vi "LvMPDC_CMD_Playlist_delete.vi"(6 "timeout_ms":i32=3000, 8 "error in (no error)":errorcluster, 9 "ReadBytes":i32=1024, 10 "pos":i32=-1, 11 "Connect ID":refnum<k5>) -> (0 "error out":errorcluster, 3 "Connect ID out":refnum<k5>)   [LabVIEW 2012]
panel:
  # "LvMPDC:: CMD delete (delete from Playlist)"
  # "-1 は番号指定無し"
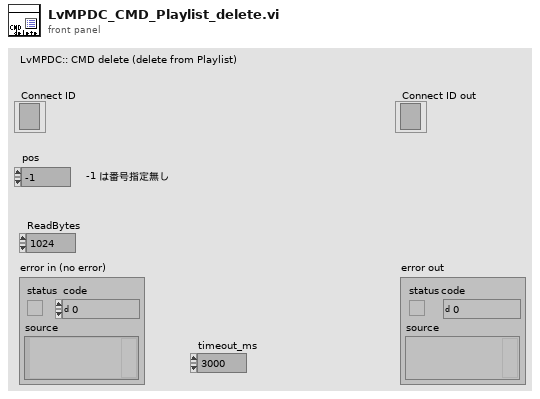
[diagram p1: front panel]
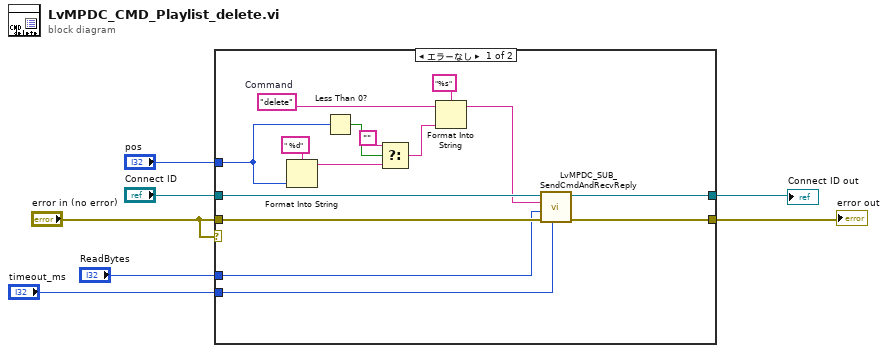
[diagram p0: block diagram]
diagram:
  n1 = case shown="エラーなし" "error in (no error)" {
    tunnel: "Connect ID" -> [w20 w24]
    tunnel: "error in (no error)" -> [w22 w23]
    tunnel: [w19 w24] -> w6
    tunnel: [w21 w23] -> w5
    tunnel: "timeout_ms" -> [w17 _]
    tunnel: "ReadBytes" -> [w18 _]
    tunnel: "pos" -> [w13 _]
    frame No Error {
      w16 = "delete"  # Command
      n2 = Format Into String(format string=" %d" ("形式文字列"), w13) -> (resulting string=w10:string)  [unwired: 2 in, 1 out]
      n3 = Less Than 0?(x=w13) -> (x < 0?=w12:bool)
      n4 = Select(t="", s=w12, f=w10) -> (s? t:f=w9:string)
      n5 = Format Into String(format string="%s" ("形式文字列"), initial string=w16, w9) -> (resulting string=w8:string)  [unwired: 1 in, 1 out]
      n6 = call "LvMPDC_SUB_SendCmdAndRecvReply.vi"("timeout_ms"=w17, "error in (no error)"=w22, "ReadBytes"=w18, "Command"=w8, "Connect ID"=w20) -> ("error out"=w21:errorcluster, "Connect ID out"=w19:refnum<k5>)  [unwired: 4 in, 1 out]
    }
    frame Error {
    }
  }
  "Connect ID out" <- w6
  "error out" <- w5
